vi "Do.vi"(8 "error in (no error)":errorcluster, 10 "Actor in":refnum<class "Actor.lvclass">, 11 "Launch Workers Msg":refnum<class "Launch Reader Msg.lvclass">) -> (0 "error out":errorcluster, 2 "Actor out":refnum<class "Actor.lvclass">)   [LabVIEW 2020, in "ConnectionManager.lvlib" / "Launch Reader Msg.lvclass"]
doc: "This VI delivers the message to the actor by calling the appropriate method(s) on the actor."
uses:
  <vilib>/gpm_packages/@cs/Network-interface/Source/ConnectionManager/ConnectionManager Messages/Launch Reader Msg/Launch Reader Msg.lvclass
  <vilib>/ActorFramework/Actor/Actor.lvclass
  <vilib>/gpm_packages/@cs/Network-interface/Source/ConnectionManager/ConnectionManager/ConnectionManager.lvclass
  C:/Program Files/National Instruments/LabVIEW 2020/vi.lib/ActorFramework/Actor/Actor.lvclass
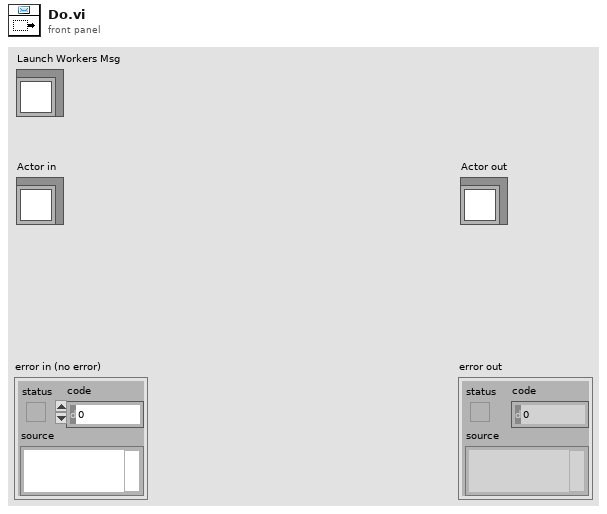
[diagram p1: front panel]
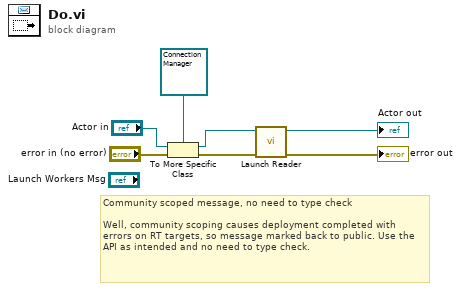
[diagram p0: block diagram]
diagram:
  # "Community scoped message, no need to type check\n\nWell, community scoping causes deployment completed with errors on RT targets, so message marked back to public. Use the API as intended and no need to type check."
  n1 = To More Specific Class(target class=refnum<class "ConnectionManager.lvclass"> refnum ("Actor in"), reference="Actor in", error in="error in (no error)") -> (specific class reference=w1:refnum<class "ConnectionManager.lvclass">, error out=w6:errorcluster)
  n2 = call <vilib>:"Launch Reader.vi"("error in (no error)"=w6, "ConnectionManager in"=w1) -> ("error out"=→"error out":errorcluster, "ConnectionManager out"=→"Actor out":refnum<class "ConnectionManager.lvclass">)  [unwired: 8 in]
